vi "Delete String Array Element.vi"(10 "Element to Delete":string, 11 "Array in":string[](array[string])) -> (2 "Found and Deleted":bool, 3 "Array out":string[](array[string]))   [LabVIEW 2020, in "Wordle Engine.lvlib"]
uses:
  Wordle Engine.lvlib
  fe6ff793-1998-4283-98d7-6c1f135b3a18.vi
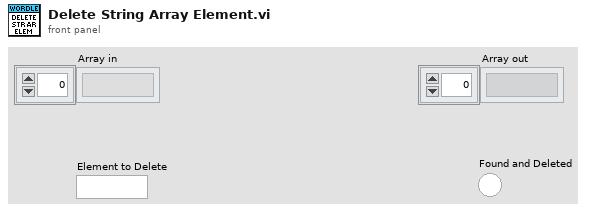
[diagram p1: front panel]
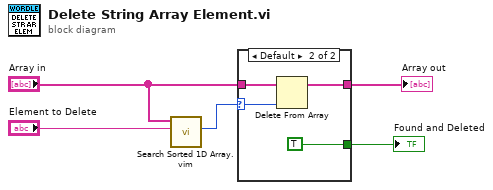
[diagram p0: block diagram]
diagram:
  n1 = call "Search Sorted 1D Array.vim"("element"="Element to Delete", "sorted 1D array"="Array in") -> ("nearest index"=w5:i32)  [unwired: 8 in, 1 out]
  n2 = case shown="Default" w5 {
    selector: w5 -> [_ w10]
    tunnel: "Array in" -> [w6 w9]
    tunnel: [w6 w8] -> w2
    tunnel: [_ TRUE] -> w1
    frame -1 {
    }
    frame Default {
      n3 = Delete From Array(array=w9, index=w10) -> (array with subset deleted=w8:string[])  [unwired: 1 in, 1 out]
    }
  }
  "Array out" <- w2
  "Found and Deleted" <- w1
